vi "Close.vi"(8 "error in (no error)":errorcluster, 11 "Relay-Box in":refnum<class "Relay-Box.lvclass">) -> (0 "error out":errorcluster, 2 "FT_Status":u32(ring) items=["FT_OK", "FT_INVALID_HANDLE", "FT_DEVICE_NOT_FOUND", "FT_DEVICE_NOT_OPENED", "FT_IO_ERROR", "FT_INSUFFICIENT_RESOURCES", "FT_INVALID_PARAMETER", "FT_INVALID_BAUD_RATE", "FT_DEVICE_NOT_OPENED_FOR_ERASE", "FT_DEVICE_NOT_OPENED_FOR_WRITE", "FT_FAILED_TO_WRITE_DEVICE", "FT_EEPROM_READ_FAILED", "FT_EEPROM_WRITE_FAILED", "FT_EEPROM_ERASE_FAILED", "FT_EEPROM_NOT_PRESENT", "FT_EEPROM_NOT_PROGRAMMED", "FT_INVALID_ARGS", "FT_NOT_SUPPORTED", "FT_OTHER_ERROR"], 3 "Relay-Box out":refnum<class "Relay-Box.lvclass">)   [LabVIEW 2019, in "Relay-Box.lvclass"]
uses:
  <userlib>/LevyLab/Relay Box/Relay-Box.lvclass
  <userlib>/LevyLab/Relay Box/Relay-Box.lvclass/Relay-Box.ctl
  <userlib>/LevyLab/Relay Box/D2XX_Functions/D2XX_Functions.lvlib
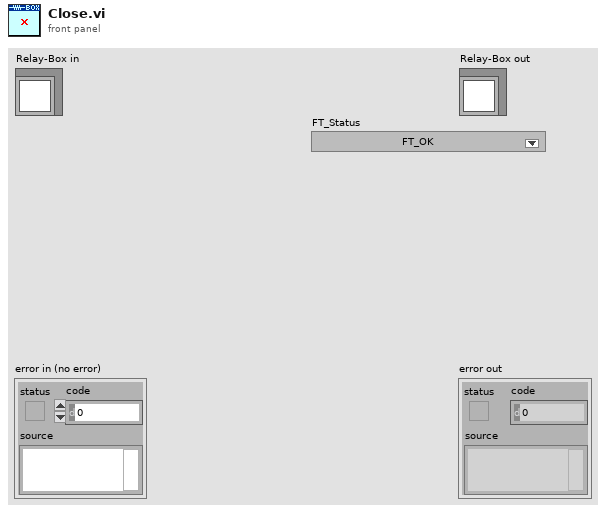
[diagram p1: front panel]
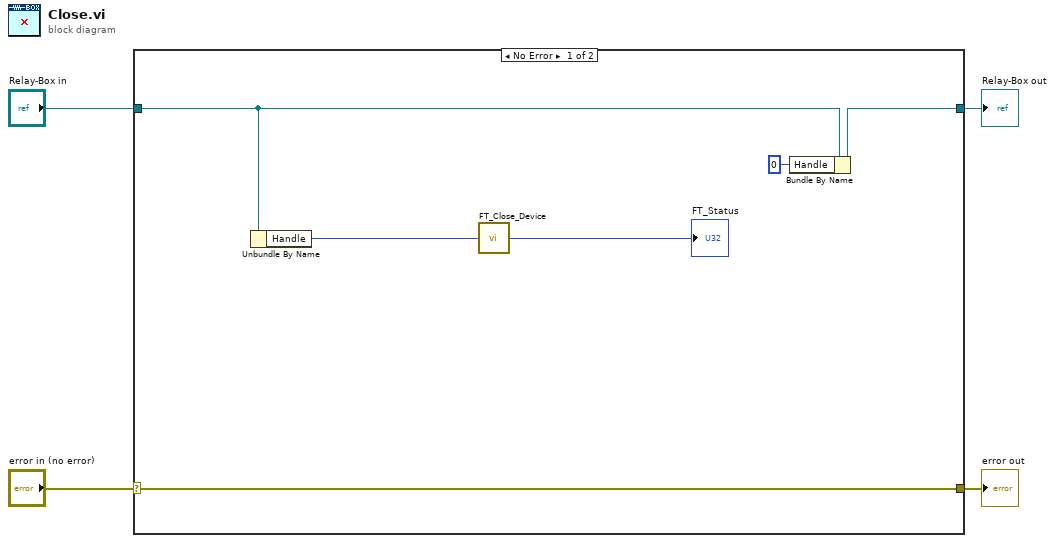
[diagram p0: block diagram]
diagram:
  n1 = case shown="No Error" "error in (no error)" {
    selector: "error in (no error)" -> [w9 w12]
    tunnel: [w9 w12] -> w3
    tunnel: [w10 w11] -> w1
    tunnel: "Relay-Box in" -> [w8 w11]
    frame No Error {
      n2 = Unbundle By Name(w8) -> ("Handle"=w7:u32)
      n3 = call <userlib>:"FT_Close_Device.vi"("Handle"=w7) -> ("FT_Status"=→"FT_Status":u32)
      n4 = Bundle By Name(cluster=w8, "Handle"=u32 0) -> (w10:refnum<class "Relay-Box.lvclass">)
    }
    frame Error {
    }
  }
  "error out" <- w3
  "Relay-Box out" <- w1
